vi "Get Samples Per Second from NI 9234 Configuration.vi"(4 "Sample Rate (51.2k )":T1=1 caption="采样率(51.2k)" items=["51.200 kS/s (NI 9234)"=1, "25.600 kS/s (NI 9234)"=2, "17.067 kS/s (NI 9234)"=3, "12.800 kS/s (NI 9234)"=4, "10.240 kS/s (NI 9234)"=5, "8.533 kS/s (NI 9234)"=6, "7.314 kS/s (NI 9234)"=7, "6.400 kS/s (NI 9234)"=8, "5.689 kS/s (NI 9234)"=9, "5.120 kS/s (NI 9234)"=10, "4.654 kS/s (NI 9234)"=11, "4.267 kS/s (NI 9234)"=12, "3.938 kS/s (NI 9234)"=13, "3.657 kS/s (NI 9234)"=14, "3.413 kS/s (NI 9234)"=15, "3.200 kS/s (NI 9234)"=16, "3.012 kS/s (NI 9234)"=17, "2.845 kS/s (NI 9234)"=18, "2.695 kS/s (NI 9234)"=19, "2.560 kS/s (NI 9234)"=20, "2.438 kS/s (NI 9234)"=21, "2.328 kS/s (NI 9234)"=22, "2.226 kS/s (NI 9234)"=23, "2.133 kS/s (NI 9234)"=24, "2.048 kS/s (NI 9234)"=25, "1.969 kS/s (NI 9234)"=26, "1.896 kS/s (NI 9234)"=27, "1.829 kS/s (NI 9234)"=28, "1.765 kS/s (NI 9234)"=29, "1.707 kS/s (NI 9234)"=30, "1.652 kS/s (NI 9234)"=31]) -> (1 "Samples per second":dbl caption="每秒采样数")   [LabVIEW 2013]
uses:
  <vilib>/LabVIEW Targets/FPGA/cRIO/shared/nicrio_ModuleControls/nicrio_cRIO-9234_DataRatesRing2.ctl
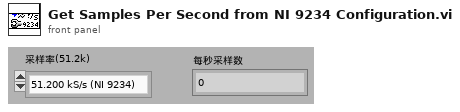
[diagram p1: front panel]
types:
  T1 = typedef "nicrio_cRIO-9234_DataRatesRing2.ctl" = u8
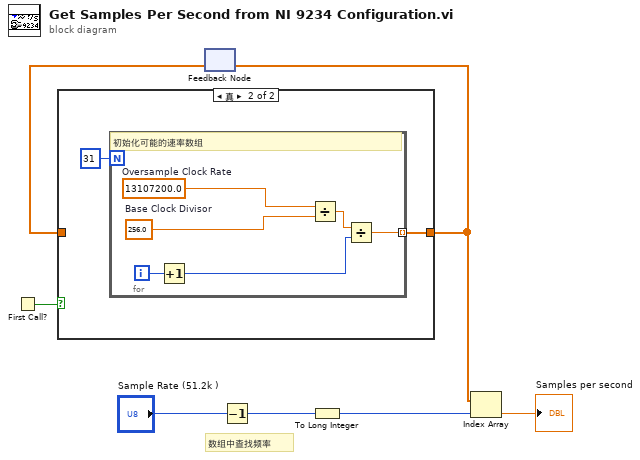
[diagram p0: block diagram]
diagram:
  # "数组中查找频率"
  n1 = First Call?() -> (First Call?: T/F=w4:bool)
  n2 = feedback #1() -> (w2:dbl[])  [unwired: 1 in]
  n3 = case shown="真" w4 {
    tunnel: [w8 w9] -> w3
    tunnel: w2 -> [w8 _]
    frame False {
    }
    frame True {
      n4 = for {
        N: 31 -> [_]
        tunnel: [w11] -> w9 mode=indexing
        i -> [w16]
        w14 = 256.0  # Base Clock Divisor
        w15 = 13107200.0  # Oversample Clock Rate
        # "初始化可能的速率数组"
        n5 = Increment(x=w16) -> (x+1=w12:i32)
        n6 = Divide(x=w15, y=w14) -> (x/y=w13:dbl)
        n7 = Divide(x=w13, y=w12) -> (x/y=w11:dbl)
      }
    }
  }
  n8 = feedback-in #1(w3) -> ()
  n9 = Decrement(x="Sample Rate (51.2k )") -> (x-1=w5:T1)
  n10 = To Long Integer(number=w5) -> (32bit integer=w7:i32)
  n11 = Index Array(array=w3, index=w7) -> (element=→"Samples per second":dbl)
